vi "Get MAX position.vi"(0 "Zaber":T1={"Serial port handle"="", "Axis"="", "Controller #"=0, "Min position"=0.0, "Max position"=0.0, "Min velocity"=0.0, "Max velocity"=0.0, "Firmware"="", "Device ID"=0, "Variable event"=refnum, "Variable ref"=refnum, "Resolution, usteps/step"=0, "Serial port semaphore"=refnum, "Joystick buttons"={"MinDir"=1, "MaxDir"=2, "MedSpeed"=5, "HighSpeed"=6}} {"Joystick buttons"."HighSpeed" min=1 max=25 step=1; "Joystick buttons"."MedSpeed" min=1 max=25 step=1; "Joystick buttons"."MaxDir" min=1 max=25 step=1; "Joystick buttons"."MinDir" min=1 max=25 step=1}, 5 "error in":errorcluster) -> (14 "Zaber out":T1={"Serial port handle"="", "Axis"="", "Controller #"=0, "Min position"=0.0, "Max position"=0.0, "Min velocity"=0.0, "Max velocity"=0.0, "Firmware"="", "Device ID"=0, "Variable event"=refnum, "Variable ref"=refnum, "Resolution, usteps/step"=0, "Serial port semaphore"=refnum, "Joystick buttons"={"MinDir"=1, "MaxDir"=2, "MedSpeed"=5, "HighSpeed"=6}} {"Joystick buttons"."HighSpeed" min=1 max=25 step=1; "Joystick buttons"."MedSpeed" min=1 max=25 step=1; "Joystick buttons"."MaxDir" min=1 max=25 step=1; "Joystick buttons"."MinDir" min=1 max=25 step=1}, 16 "MAX position, mm":dbl, 17 "MAX position, usteps":i32, 19 "error out":errorcluster)   [LabVIEW 2018]
uses:
  Zaber.ctl
  GenericDataEvent/GenericEvent.ctl
  ZaberVariables.ctl
  CommandZaber.ctl
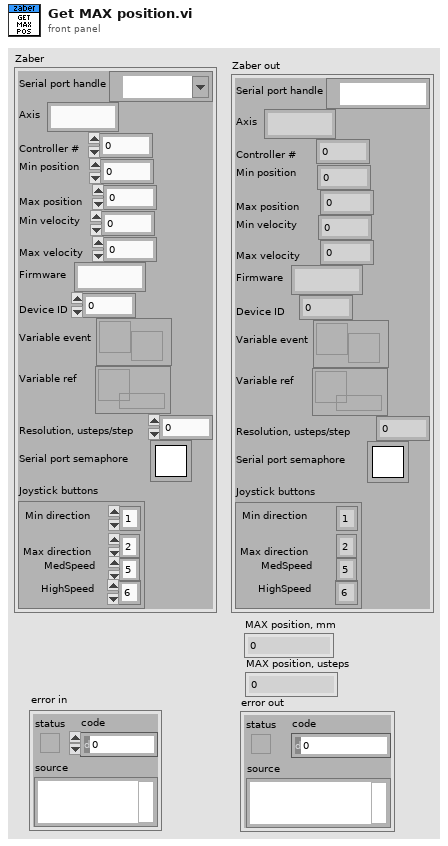
[diagram p1: front panel]
types:
  T1 = typedef "Zaber.ctl" = cluster{"Serial port handle":refnum<visa-resource-name>, "Axis":string, "Controller #":u8, "Min position":dbl, "Max position":dbl, "Min velocity":dbl, "Max velocity":dbl, "Firmware":string, "Device ID":i32, "Variable event":T2, "Variable ref":refnum<data-value>, "Resolution, usteps/step":i32, "Serial port semaphore":T3, "Joystick buttons":cluster{"MinDir":i32, "MaxDir":i32, "MedSpeed":i32, "HighSpeed":i32}}
  T2 = typedef "GenericEvent.ctl" = refnum<user-event>
  T3 = typedef "Semaphore RefNum" = refnum<k1>
  T4 = typedef "CommandZaber.ctl" = cluster{"Command":u8, "Data":i32}
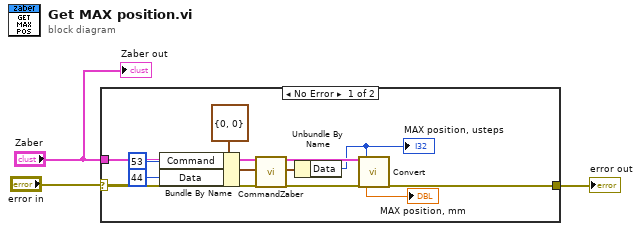
[diagram p0: block diagram]
diagram:
  n1 = case shown="No Error" "error in" {
    selector: "error in" -> [w11 w16]
    tunnel: [w4 w16] -> w1
    tunnel: "Zaber" -> [w10 _]
    frame No Error {
      n2 = Bundle By Name(cluster=T4 {"Command"=0, "Data"=0} ("Command"), "Command"=53 ("Data"), "Data"=44) -> (w13:T4)
      n3 = call "CommandZaber.vi"("Zaber"=w10, "Command"=w13, "error in"=w11) -> ("Zaber out"=w8:T1, "Answer"=w9:T4, "error out"=w5:errorcluster)  [unwired: 13 in, 1 out]
      n4 = Unbundle By Name(w9) -> ("Data"=w7:i32)
      "MAX position, usteps" <- w7
      n5 = call "Convert.vi"("Zaber"=w8, "error in"=w5, "Position, usteps"=w7) -> ("Position, mm"=→"MAX position, mm":dbl, "error out"=w4:errorcluster)  [unwired: 8 in, 7 out]
    }
    frame Error {
    }
  }
  "error out" <- w1
  "Zaber out" <- "Zaber"
